vi "Read Loop Async.vi"(11 "Endpoint in":refnum<class "Endpoint.lvclass">) -> ()   [LabVIEW 2020, in "Stream-Simple-Msg.lvlib" / "Endpoint.lvclass"]
uses:
  Endpoint.lvclass
  Endpoint.lvclass/Endpoint.ctl
  <vilib>/IlluminatedG/lv-stream/stream/Stream.lvclass
  Manager/Manager.lvclass
  Message/Message.lvclass
  <vilib>/IlluminatedG/lv-stream/URI/URI.lvclass
panel:
  out "URI String":string
  out "Raw":string
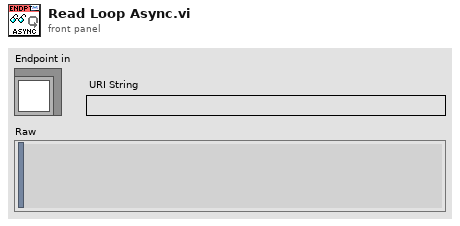
[diagram p1: front panel]
types:
  T1 = typedef "Stream.lvlib/Flatten Type.ctl" = enum16{"String", "JSON", "Custom"}
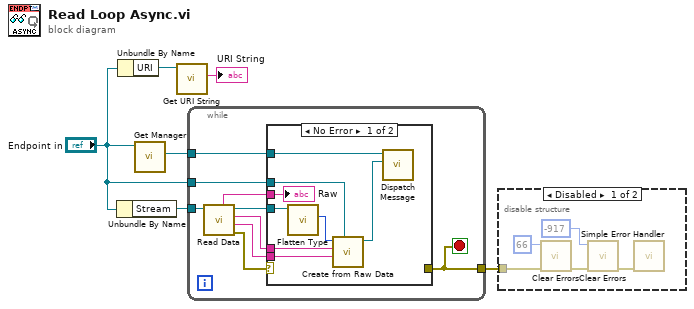
[diagram p0: block diagram]
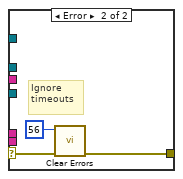
[diagram p3: hidden frame]
diagram:
  n1 = Unbundle By Name("Endpoint in") -> ("Stream"=w6:refnum<class "Stream.lvclass">)
  n2 = Unbundle By Name("Endpoint in") -> ("URI"=w2:refnum<class "URI.lvclass">)
  n3 = call "Get Manager.vi"("Endpoint in"="Endpoint in") -> ("Manager"=w5:refnum<class "Manager.lvclass">)  [unwired: 8 in, 2 out]
  n4 = call <vilib>:"Get URI String.vi"("URI in"=w2) -> ("URI String"=→"URI String":string)  [unwired: 8 in, 2 out]
  n5 = while {
    tunnel: w6 -> [w12]
    tunnel: w5 -> [w15]
    tunnel: "Endpoint in" -> [w14]
    tunnel: [w13] -> w4
    stop <- w13 stop-if-true
    n6 = call <vilib>:"Read Data.vi"("Stream in"=w12) -> ("error out"=w11:errorcluster, "ID (Messages)"=w10:string, "Data"=w9:string, "Stream out"=w8:refnum<class "Stream.lvclass">, "Raw"=w7:string)  [unwired: 6 in]
    n7 = case shown="No Error" w11 {
      selector: w11 -> [_ w26]
      tunnel: w15 -> [w23 _]
      tunnel: w14 -> [w22 _]
      tunnel: [_ w24] -> w13
      tunnel: w9 -> [w18 _]
      tunnel: w10 -> [w19 _]
      tunnel: w8 -> [w20 _]
      tunnel: w7 -> [w16 _]
      frame No Error {
        n8 = call-dynamic "Flatten Type.vi"("Stream in"=w20) -> ("Flatten Type"=w17:T1)  [unwired: 8 in, 2 out]
        n9 = call "Create from Raw Data.vi"("Endpoint"=w22, "ID"=w19, "Raw Data"=w18, "Flatten Type"=w17) -> ("Message out"=w21:refnum<class "Message.lvclass">)  [unwired: 6 in, 1 out]
        n10 = call "Dispatch Message.vi"("Message"=w21, "Manager in"=w23) -> ()  [unwired: 8 in, 2 out]
        "Raw" <- w16
      }
      frame Error {
        # "Ignore timeouts"
        n11 = call <vilib>:"Clear Errors.vi"("error in (no error)"=w26, "specific error code to clear (0: all)"=56) -> ("error out"=w24:errorcluster)  [unwired: 4 in, 1 out]
      }
    }
  }
  n12 = disable-structure shown="Disabled" {
    disable-tunnel: w4 -> [w31 _]
    frame Disabled {
      n13 = call <vilib>:"Clear Errors.vi"("error in (no error)"=w31, "specific error code to clear (0: all)"=66) -> ("error out"=w29:errorcluster)  [unwired: 4 in, 1 out]
      n14 = call <vilib>:"Clear Errors.vi"("error in (no error)"=w29, "specific error code to clear (0: all)"=-917) -> ("error out"=w27:errorcluster)  [unwired: 4 in, 1 out]
      n15 = call <vilib>:"Simple Error Handler.vi"("error in (no error)"=w27) -> ()  [unwired: 4 in, 5 out]
    }
    frame Enabled {
    }
  }
